vi "Sub1.vi"(8 "error in (no error)":errorcluster, 9 "URL":string) -> (0 "error out":errorcluster, 10 "ISS Lat":dbl, 11 "ISS Lon":dbl)   [LabVIEW 2018]
doc: "Use this template to build a VI to use as a subVI. This subVi with error handler contacts the web server and reads the result. Get this information from the web server and display your own world map in LabVIEW with the current position of the ISS."
uses:
  <vilib>/Utility/error.llb/Error Cluster From Error Code.vi
  <vilib>/ErrorRing/Error Ring.xnode
  <vilib>/httpClient/LabVIEWHTTPClient.lvlib
panel:
  out "A * B":dbl
  out "number 2":dbl
  out "number":dbl
  out "substring 2":string
  out "substring":string
  out "after substring 2":string
  out "after substring":string
  out "body":string
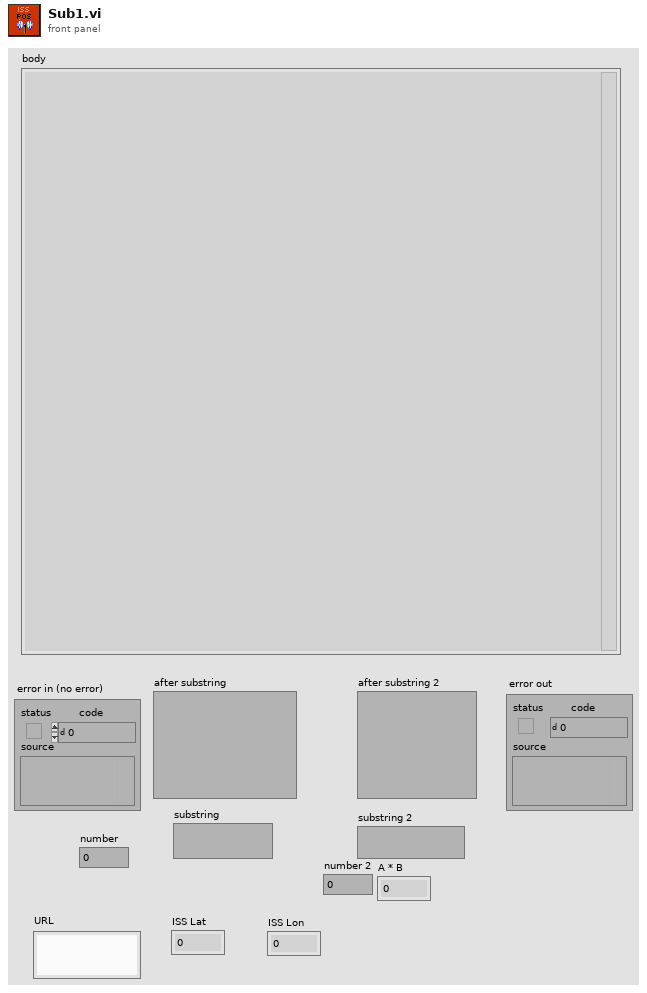
[diagram p1: front panel]
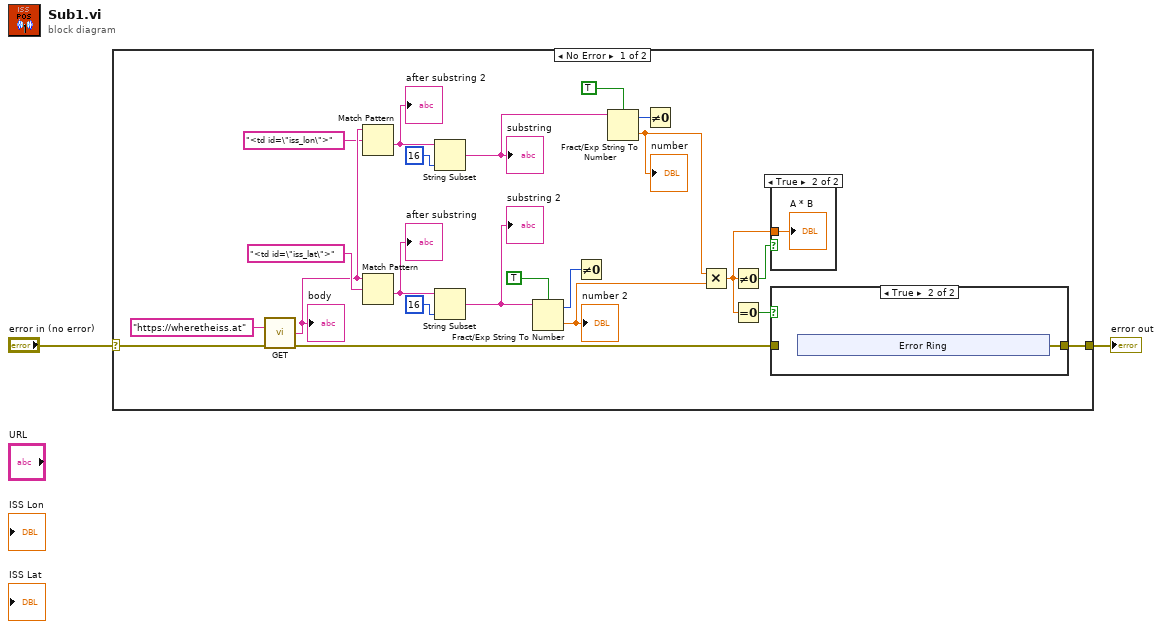
[diagram p0: block diagram]
diagram:
  n1 = case shown="No Error" "error in (no error)" {
    selector: "error in (no error)" -> [w23 w33]
    tunnel: [w3 w33] -> w1
    frame No Error {
      n2 = call <vilib>:"GET.vi"("url"="https://wheretheiss.at", "error in (no error)"=w23) -> ("body"=w21:string, "error out"=w4:errorcluster)  [unwired: 10 in, 2 out]
      "body" <- w21
      n3 = Match Pattern(string=w21, regular expression="<td id=\"iss_lon\">") -> (after substring=w19:string)  [unwired: 1 in, 3 out]
      "after substring 2" <- w19
      n4 = Match Pattern(string=w21, regular expression="<td id=\"iss_lat\">") -> (after substring=w17:string)  [unwired: 1 in, 3 out]
      "after substring" <- w17
      n5 = String Subset(string=w19, length (rest)=16 ("length (rest)")) -> (substring=w12:string)  [unwired: 1 in]
      "substring" <- w12
      n6 = String Subset(string=w17, length (rest)=16 ("length (rest)")) -> (substring=w14:string)  [unwired: 1 in]
      "substring 2" <- w14
      n7 = Fract/Exp String To Number(use system decimal point (T)=TRUE, string=w14) -> (offset past number=w10:i32, number=w8:dbl)  [unwired: 2 in]
      "number 2" <- w8
      n8 = Not Equal To 0?(x=w10) -> ()  [unwired: 1 out]
      n9 = Fract/Exp String To Number(use system decimal point (T)=TRUE, string=w12) -> (offset past number=w11:i32, number=w9:dbl)  [unwired: 2 in]
      "number" <- w9
      n10 = Not Equal To 0?(x=w11) -> ()  [unwired: 1 out]
      n11 = Multiply(x=w9, y=w8) -> (x*y=w5:dbl)
      n12 = Not Equal To 0?(x=w5) -> (x != 0?=w6:bool)
      n13 = Equal To 0?(x=w5) -> (x = 0?=w7:bool)
      n14 = case shown="True" w6 {
        tunnel: w5 -> [_ w25]
        frame False {
        }
        frame True {
          "A * B" <- w25
        }
      }
      n15 = case shown="True" w7 {
        tunnel: w4 -> [w26 _]
        tunnel: [w26 w27] -> w3
        frame False {
        }
        frame True {
          n16 = xnode "Error Ring"() -> ("error out"=w27:errorcluster)
        }
      }
    }
    frame Error {
    }
  }
  "error out" <- w1
